vi "attach_listener.vi"(8 "error in (no error)":errorcluster, 9 "type":T1, 10 "listener":refnum<class "GenericToplevelComponent.lvclass">, 11 "GenericImageAssembler in":refnum<class "GenericImageAssembler.lvclass">) -> (0 "error out":errorcluster, 3 "GenericImageAssembler out":refnum<class "GenericImageAssembler.lvclass">)   [LabVIEW 2010]
uses:
  common/classes/ErrorController/ErrorController/ErrorController.lvclass
  type_enum.ctl
  GenericImageAssembler.lvclass
  listener_cluster.ctl
  common/classes/GenericToplevelComponent/GenericToplevelComponent/GenericToplevelComponent.lvclass
  common/classes/GenericComponent/GenericComponent/GenericComponent.lvclass
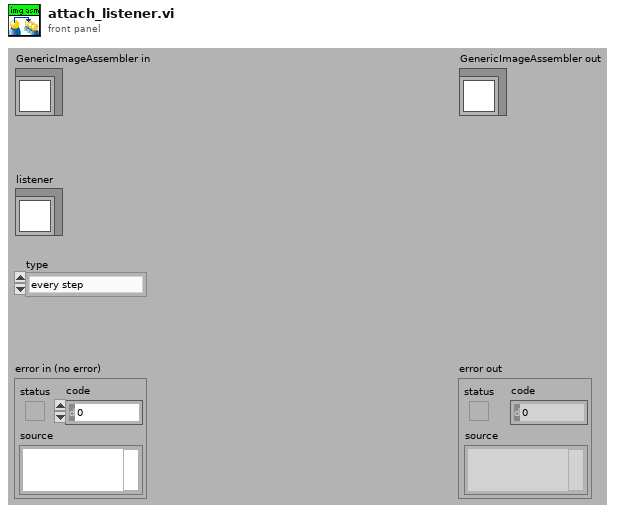
[diagram p1: front panel]
types:
  T1 = typedef "GenericImageAssembler.lvclass/type_enum.ctl" = enum16{"every step", "finalised images"}
  T2 = typedef "GenericImageAssembler.lvclass/listener_cluster.ctl" = cluster{"component":refnum<class "GenericToplevelComponent.lvclass">, "type":T1}
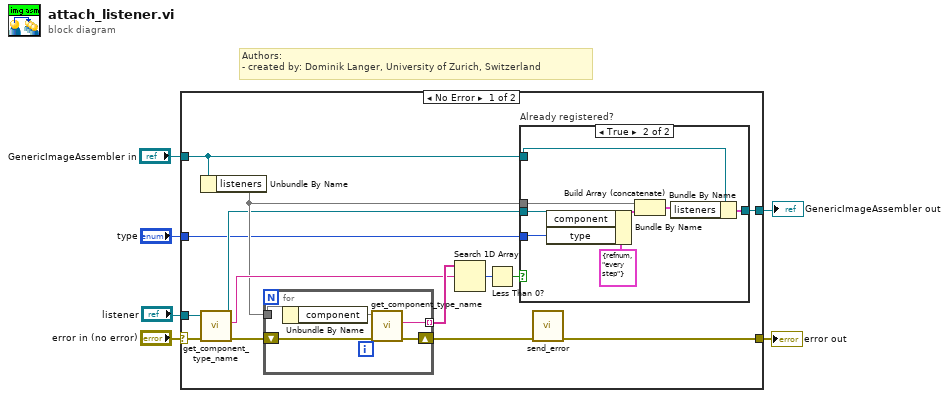
[diagram p0: block diagram]
diagram:
  # "Authors: \n- created by: Dominik Langer, University of Zurich, Switzerland"
  n1 = case shown="No Error" "error in (no error)" {
    selector: "error in (no error)" -> [w20 w36]
    tunnel: [w8 w36] -> w2
    tunnel: [w11 w35] -> w3
    tunnel: "GenericImageAssembler in" -> [w10 w35]
    tunnel: "listener" -> [w18 _]
    tunnel: "type" -> [w7 _]
    frame No Error {
      n2 = Unbundle By Name(w10) -> ("listeners"=w13)
      n3 = call-dynamic "get_component_type_name.vi"("error in (no error)"=w20, "GenericPlugin in"=w18) -> ("error out"=w19:errorcluster, "component type"=w16:string, "GenericPlugin out"=w12:refnum<class "GenericToplevelComponent.lvclass">)  [unwired: 7 in]
      n4 = for {
        shift-right: [w33] -> w9
        shift-left: w19 -> [w34]
        tunnel: w13 -> [w30]
        tunnel: [w32] -> w17 mode=indexing
        n5 = Unbundle By Name(w30) -> ("component"=w31)
        n6 = call-dynamic "get_component_type_name.vi"("error in (no error)"=w34, "GenericPlugin in"=w31) -> ("error out"=w33:errorcluster, "component type"=w32:string)  [unwired: 7 in, 1 out]
      }
      n7 = Search 1D Array(1D array=w17, element=w16) -> (index of element=w15:i32)  [unwired: 1 in]
      n8 = Less Than 0?(x=w15) -> (x < 0?=w14:bool)
      n9 = case "Already registered?" shown="True" w14 {
        tunnel: w13 -> [_ w29]
        tunnel: w12 -> [_ w24]
        tunnel: w10 -> [w21 w27]
        tunnel: [w21 w26] -> w11
        tunnel: w7 -> [_ w23]
        frame False {
        }
        frame True {
          n10 = Bundle By Name(cluster=T2 {"component"=refnum, "type"=enum."every step"} ("listener"), "component"=w24, "type"=w23) -> (w22:T2)
          n11 = Build Array (concatenate)(w29, w22) -> (w28:T2[])
          n12 = Bundle By Name(cluster=w27, "listeners"=w28) -> (w26:cluster{})
        }
      }
      n13 = call "send_error.vi"("error in (no error)"=w9) -> ("error out"=w8:errorcluster)  [unwired: 10 in]
    }
    frame Error {
    }
  }
  "error out" <- w2
  "GenericImageAssembler out" <- w3
